vi "Create folders on network and group server.vi"(11 "File path in":path) -> (3 "File path out":path)   [LabVIEW 2011]
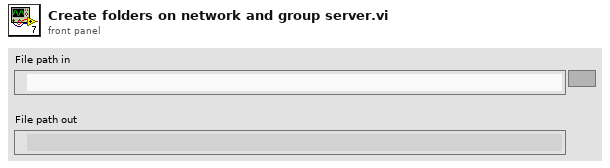
[diagram p1: front panel]
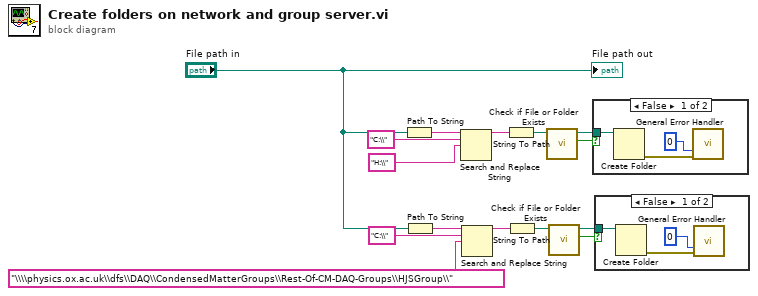
[diagram p0: block diagram]
diagram:
  n1 = Path To String(path="File path in") -> (string=w14:string)
  n2 = Path To String(path="File path in") -> (string=w10:string)
  n3 = Search and Replace String(input string=w14, search string="C:\\", replace string="H:\\") -> (result string=w15:string)  [unwired: 5 in, 3 out]
  n4 = Search and Replace String(input string=w10, search string="C:\\", replace string="\\\\physics.ox.ac.uk\\dfs\\DAQ\\CondensedMatterGroups\\Rest-Of-CM-DAQ-Groups\\HJSGroup\\") -> (result string=w11:string)  [unwired: 5 in, 3 out]
  n5 = String To Path(string=w15) -> (path=w5:path)
  n6 = String To Path(string=w11) -> (path=w2:path)
  n7 = call <vilib>:"Check if File or Folder Exists.vi"("path"=w5) -> ("file or folder exists?"=w7:bool, "dup path"=w6:path)  [unwired: 8 in, 1 out]
  n8 = call <vilib>:"Check if File or Folder Exists.vi"("path"=w2) -> ("file or folder exists?"=w4:bool, "dup path"=w3:path)  [unwired: 8 in, 1 out]
  n9 = case shown="False" w7 {
    tunnel: w6 -> [w18 _]
    frame False {
      n10 = Create Folder(path (use dialog)=w18) -> (error out=w17:errorcluster)  [unwired: 2 in, 2 out]
      n11 = call <vilib>:"General Error Handler.vi"("type of dialog (OK msg:1)"=0, "error in (no error)"=w17) -> ()  [unwired: 9 in, 5 out]
    }
    frame True {
    }
  }
  n12 = case shown="False" w4 {
    tunnel: w3 -> [w21 _]
    frame False {
      n13 = Create Folder(path (use dialog)=w21) -> (error out=w20:errorcluster)  [unwired: 2 in, 2 out]
      n14 = call <vilib>:"General Error Handler.vi"("type of dialog (OK msg:1)"=0, "error in (no error)"=w20) -> ()  [unwired: 9 in, 5 out]
    }
    frame True {
    }
  }
  "File path out" <- "File path in"
